vi "Begin.vi"() -> (0 "error out":errorcluster)   [LabVIEW 2011]
doc: "Called before other user functions, this VI is expected to open initial I/O refnums, load in file data, and do all program initialization. Notice that the <B>error out</B> terminal is simply used for data flow. Wiring it to other structures or subVIs ensures that this VI runs first."
uses:
  <vilib>/Rock Robotics/WPI/Joystick/WPI_JoystickDeviceEnum.ctl
  <vilib>/Rock Robotics/SystemInterfaces/DIO/FPGA_DIOChannel.ctl
  <vilib>/Rock Robotics/SystemInterfaces/Typedef/FPGA_TypedefDigitalModule.ctl
  <vilib>/Rock Robotics/SystemInterfaces/AI/FPGA_AIGyroChannel.ctl
  <vilib>/Rock Robotics/SystemInterfaces/DIO/FPGA_DIOPWMChannel.ctl
  <vilib>/Rock Robotics/SystemInterfaces/AI/FPGA_AIChannel.ctl
  <vilib>/Rock Robotics/SystemInterfaces/DIO/FPGA_DIORelayChannel.ctl
  <vilib>/Rock Robotics/SystemInterfaces/Typedef/FPGA_TypedefSolenoidModule.ctl
  <vilib>/Rock Robotics/WPI/Solenoid/WPI_SolenoidChannel.ctl
  <vilib>/Rock Robotics/WPI/Solenoid/WPI_SolenoidValue.ctl
  <vilib>/Rock Robotics/WPI/Relay/WPI_RelayDirection.ctl
  <vilib>/Rock Robotics/SystemInterfaces/Typedef/FPGA_TypedefAnalogModule.ctl
  <vilib>/Rock Robotics/WPI/Relay/WPI_RelayValue.ctl
  <vilib>/Rock Robotics/SystemInterfaces/Typedef/FPGA_TypedefAnalogModuleForGyro.ctl
  <vilib>/Rock Robotics/WPI/Counter/WPI_CounterOpen UpDown Mode.vi
  <vilib>/Rock Robotics/WPI/MotorControl/WPI_MotorControlOpen Victor.vi
  <vilib>/Rock Robotics/WPI/RobotDrive/WPI_RobotDriveOpen2MotorWithVictor.vi
  <vilib>/Rock Robotics/WPI/Solenoid/WPI_SolenoidSetEnum.vi
  <vilib>/Rock Robotics/WPI/Solenoid/WPI_SolenoidOpenDouble.vi
  Robot Global Data.vi
  <vilib>/Rock Robotics/WPI/Camera/WPI_CameraWhite Balance Values.ctl
  <vilib>/Rock Robotics/WPI/Camera/WPI_CameraExposure Values.ctl
  <vilib>/Rock Robotics/WPI/Camera/WPI_CameraFrameRate.ctl
  <vilib>/Rock Robotics/WPI/RobotDrive/WPI_RobotDriveOpen4MotorWithVictor.vi
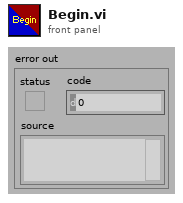
[diagram p1: front panel]
types:
  T1 = typedef "FPGA_AIGyroChannel.ctl" = enum8{"AI 1", "AI 2", "Invalid"}
  T2 = typedef "FPGA_TypedefAnalogModuleForGyro.ctl" = enum16{"Analog Module 1"}
  T3 = typedef "WPI_RelayDirection.ctl" = enum16{"Both directions", "Forward only", "Reverse only"}
  T4 = typedef "WPI_RelayValue.ctl" = enum16{"Off", "On", "Forward", "Reverse"}
  T5 = typedef "FPGA_DIORelayChannel.ctl" = enum8{"Relay 1", "Relay 2", "Relay 3", "Relay 4", "Relay 5", "Relay 6", "Relay 7", "Relay 8", "Invalid"}
  T6 = typedef "FPGA_TypedefDigitalModule.ctl" = enum16{"Digital Module 1", "Digital Module 2"}
  T7 = typedef "FPGA_AIChannel.ctl" = enum8{"AI 1", "AI 2", "AI 3", "AI 4", "AI 5", "AI 6", "AI 7", "AI 8", "Invalid"}
  T8 = typedef "FPGA_TypedefAnalogModule.ctl" = enum16{"Analog Module 1", "Analog Module 2"}
  T9 = typedef "FPGA_DIOPWMChannel.ctl" = enum8{"PWM 1", "PWM 2", "PWM 3", "PWM 4", "PWM 5", "PWM 6", "PWM 7", "PWM 8", "PWM 9", "PWM 10", "Invalid"}
  T10 = typedef "FPGA_DIOChannel.ctl" = enum8{"DIO 1", "DIO 2", "DIO 3", "DIO 4", "DIO 5", "DIO 6", "DIO 7", "DIO 8", "DIO 9", "DIO 10", "DIO 11", "DIO 12", "DIO 13", "DIO 14", "Invalid"}
  T11 = typedef "WPI_SolenoidValue.ctl" = enum16{"Off", "On", "Forward", "Reverse"}
  T12 = typedef "WPI_SolenoidChannel.ctl" = enum8{"Solenoid 1", "Solenoid 2", "Solenoid 3", "Solenoid 4", "Solenoid 5", "Solenoid 6", "Solenoid 7", "Solenoid 8", "Invalid"}
  T13 = typedef "FPGA_TypedefSolenoidModule.ctl" = enum16{"Solenoid Module 1", "Solenoid Module 2"}
  T14 = enum16{"Rising Edge", "Falling Edge", "Raising & Falling Edge", "Disabled"}
  T15 = typedef "WPI_JoystickDeviceEnum.ctl" = enum16{"USB 1", "USB 2", "USB 3", "USB 4", "Kinect 1", "Kinect 2"}
  T16 = typedef "WPI_CameraFrameRate.ctl" = u32
  T17 = typedef "WPI_CameraExposure Values.ctl" = enum16{"Auto", "Flicker-free 50 Hz", "Flicker-free 60 Hz", "Hold current"}
  T18 = typedef "WPI_CameraWhite Balance Values.ctl" = enum16{"Auto", "Fixed indoor", "Fixed outdoor 1", "Fixed outdoor 2", "Fixed fluorescent 1", "Fixed fluorescent 2", "Hold current"}
  T19 = typedef "WPI_CameraDevRef.ctl" = cluster{"Camera Address":string, "CameraStatus":errorcluster, "Acquire Image Notifier":refnum<notifier>}
  T20 = typedef "WPI_CameraImageSize.ctl" = enum16{"640x480", "320x240", "160x120"}
  T21 = typedef "WPI_RelayDevRef.ctl" = cluster{"DevStatus":errorcluster, "Relay Channel":T5, "Digital Module":T6, "Relay Direction":T3}
  T22 = typedef "WPI_AccelerometerDevRef.ctl" = cluster{"DevStatus":errorcluster, "Analog Module":T8, "Analog Channel":T7, "Scaling":T23}
  T23 = typedef "WPI_AccelerometerScaling.ctl" = cluster{"Gain (VoltsPerG)":dbl, "Center Voltage":dbl}
  T24 = typedef "WPI_DigitalInputDevRef.ctl" = cluster{"DevStatus":errorcluster, "DIO Channel":T10, "Digital Module":T6}
  T25 = typedef "WPI_RobotDriveDevRef.ctl" = cluster{"DevStatus":errorcluster, "Motors[]":T26[], "Square Inputs":bool, "Max Output":dbl, "Isochronous":bool}
  T26 = typedef "WPI_MotorControlDeviceRef.ctl" = cluster{"DeviceStatus":errorcluster, "Type":enum16{"PWM", "CAN"}, "PWM":cluster{"Digital Module":T6, "PWM Channel":T9, "DeadBand":T27}, "CAN":cluster{"Device Number":u8, "Control Mode":T28, "Semaphore":T29, "Max Vout":dbl}, "Invert":bool, "TransformRef":T30, "InvTransformRef":T30}
  T27 = typedef "WPI_PWMDeadband.ctl" = cluster{"Name":string, "maxPositivePwm":i32, "minPositivePwm":i32, "centerPwm":i32, "maxNegativePwm":i32, "minNegativePwm":i32, "angularRange":u16}
  T28 = typedef "WPI_CANJaguar_ControlMode.ctl" = enum8{"Percent VBus", "Current", "Speed", "Position", "Voltage"}
  T29 = typedef "Semaphore RefNum" = refnum<k1>
  T30 = typedef "WPI_PWMTransform_ConPane.ctl" = refnum<vi>
  T31 = typedef "WPI_JoystickDevRef.ctl" = cluster{"Device":T15}
  T32 = typedef "FPGA_CounterEncoderSourceConvertionLVSourceType.ctl" = cluster{"DevStatus":errorcluster, "AnalogTriggerMode?":bool, "DigitalMode":cluster{"Digital Module":T6, "DIO Channel":T33}, "AnalogTriggerMode":cluster{"AnalogTriggerIndex":T34, "OutputType":T35}}
  T33 = typedef "FPGA_DIODigitalSourceChannel.ctl" = enum8{"DIO 1", "DIO 2", "DIO 3", "DIO 4", "DIO 5", "DIO 6", "DIO 7", "DIO 8", "DIO 9", "DIO 10", "DIO 11", "DIO 12", "DIO 13", "DIO 14", "Disabled"}
  T34 = typedef "FPGA_AnalogTriggerIndex.ctl" = enum8{"Trig 0", "Trig 1", "Trig 2", "Trig 3", "Trig 4", "Trig 5", "Trig 6", "Trig 7", "Invalid"}
  T35 = typedef "FPGA_AnalogTriggerOutType.ctl" = enum16{"InWindow", "TriggerState", "Rising", "Falling"}
  T36 = typedef "WPI_AnalogChannelDevRef.ctl" = cluster{"DevStatus":errorcluster, "Analog Module":T8, "Analog Channel":T7}
  T37 = typedef "WPI_GyroDevRef.ctl" = cluster{"DevStatus":errorcluster, "Analog Module":T8, "Analog Channel":T7, "Offset":dbl, "Gain (VoltsPerDegree/Second)":dbl}
  T38 = typedef "WPI_SolenoidDevRef.ctl" = cluster{"DevStatus":errorcluster, "Solenoid Module":T13, "Forward Solenoid Channel":T12, "Reverse Solenoid Channel":T12}
  T39 = typedef "WPI_CounterDevRef.ctl" = cluster{"DevStatus":errorcluster, "CntIndex":T40}
  T40 = typedef "FPGA_CounterCtrSystemIndex.ctl" = enum8{"Ctr 0", "Ctr 1", "Ctr 2", "Ctr 3", "Ctr 4", "Ctr 5", "Ctr 6", "Ctr 7", "Invalid"}
  T41 = typedef "WPI_EncoderDevRef.ctl" = cluster{"DevStatus":errorcluster, "EncoderIndex":T42, "CounterIndex":T40, "DistancePerCount":dbl, "Decoding Type":T43}
  T42 = typedef "FPGA_EncoderIdx.ctl" = enum8{"Enc 0", "Enc 1", "Enc 2", "Enc 3", "Invalid"}
  T43 = typedef "WPI_EncoderType.ctl" = enum16{"1x", "2x", "4x"}
  T44 = typedef "WPI_ServoDeviceRef.ctl" = cluster{"DeviceStatus":errorcluster, "Digital Module":T6, "PWM Channel":T9, "DeadBand":T27}
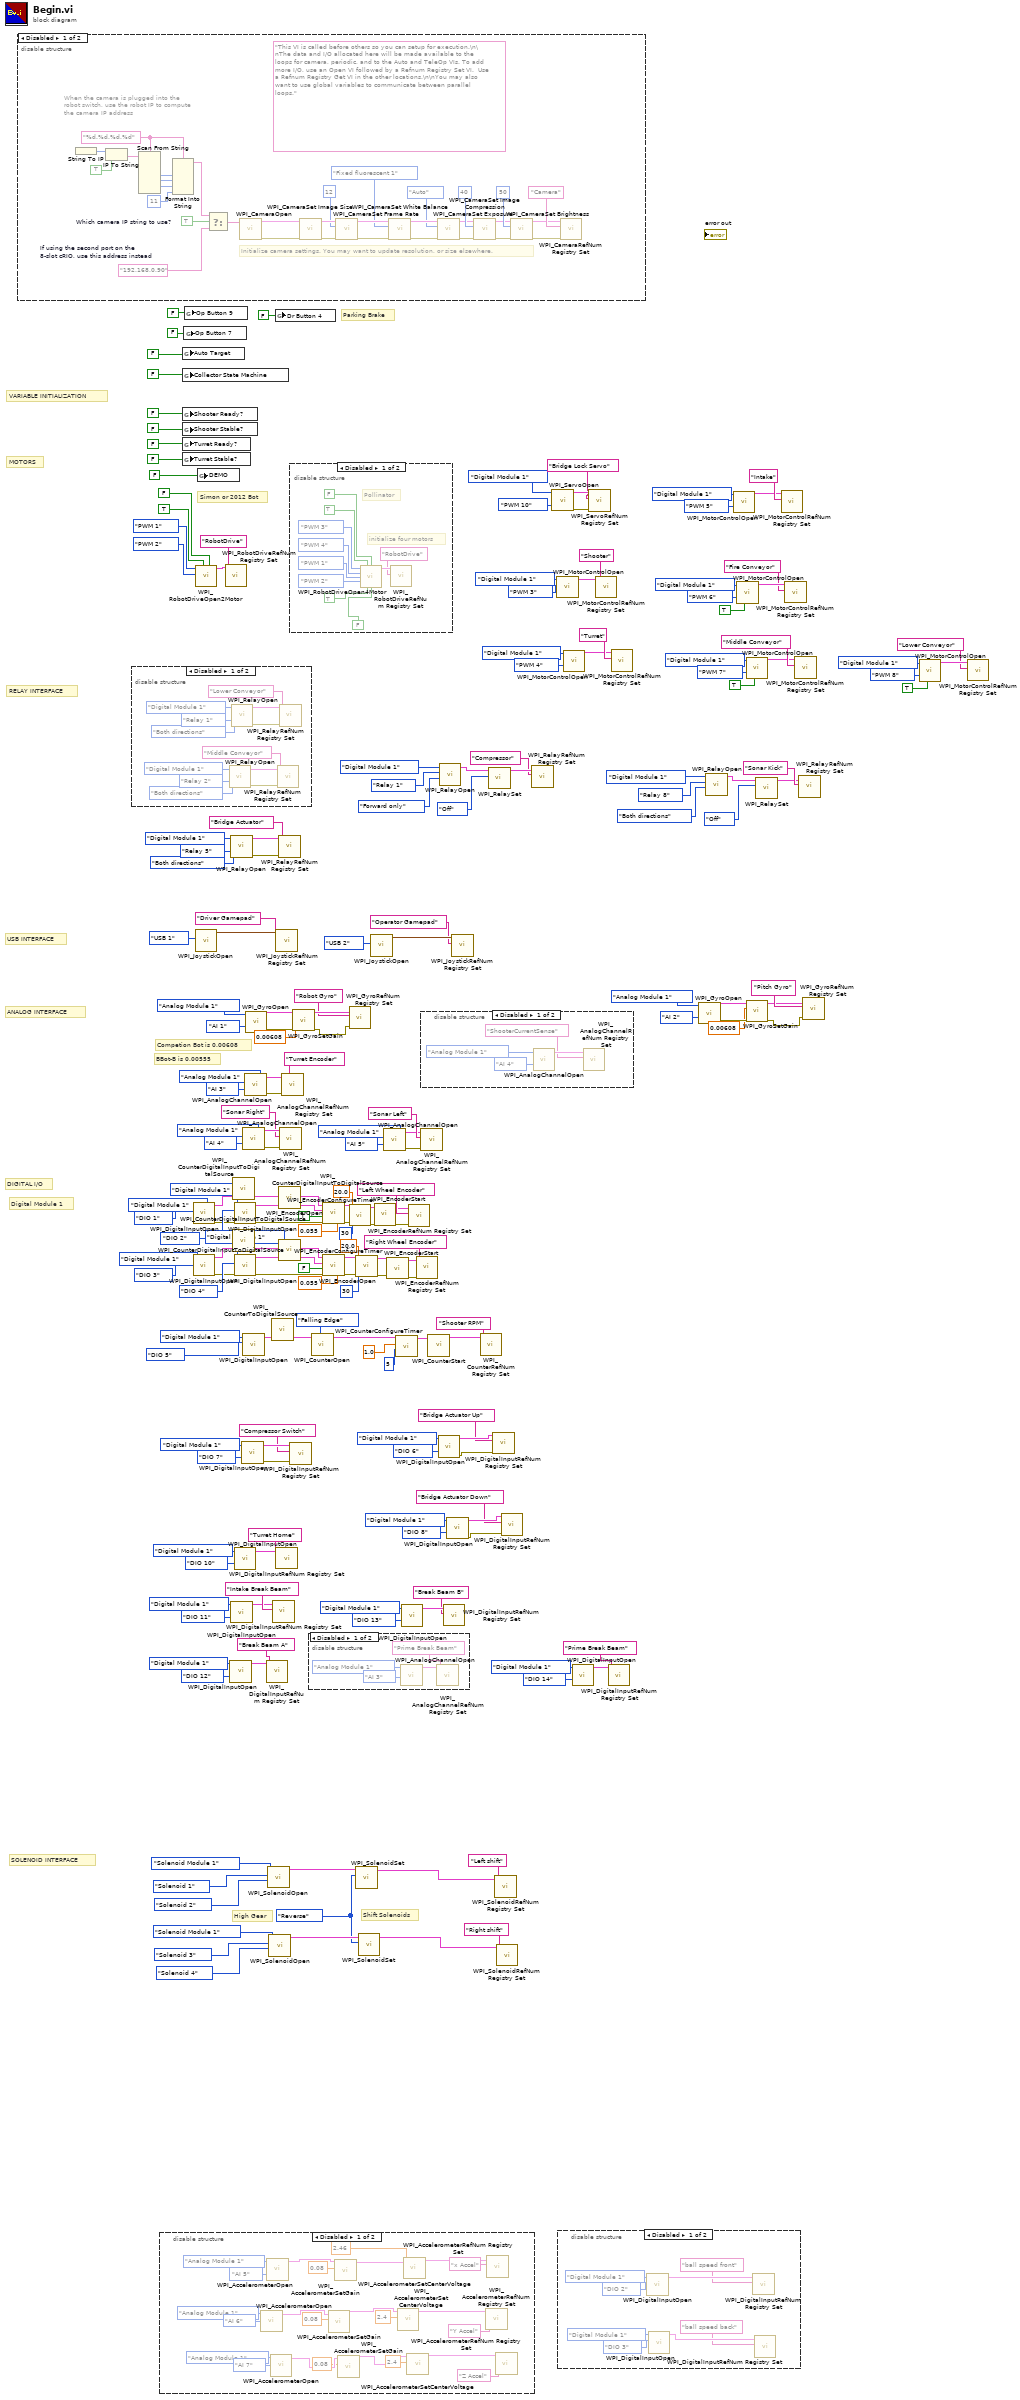
[diagram p0: block diagram]
diagram:
  w79 = WPI_SolenoidValue."Reverse" ("Value")
  # "Parking Brake"
  # "BBot-B is 0.00555"
  # "Competion Bot is 0.00608"
  # "Digital Module 1"
  # "SOLENOID INTERFACE"
  # "High Gear"
  # "Shift Solenoids"
  # "Simon or 2012 Bot"
  # "RELAY INTERFACE"
  # "MOTORS"
  # "VARIABLE INITIALIZATION"
  # "DIGITAL I/O"
  # "USB INTERFACE"
  # "ANALOG INTERFACE"
  n1 = disable-structure shown="Disabled" {
    frame Disabled {
      w207 = TRUE  # Which camera IP string to use?
      w211 = "%d.%d.%d.%d" ("format string")
      (unwired) "This VI is called before others so you can setup for execution.\n\nThe data and I/O allocated here will be made available to the loops for camera, periodic, and to the Auto and TeleOp VIs. To add more I/O, use an Open VI followed by a Refnum Registry Set VI.  Use a Refnum Registry Get VI in the other locations.\n\nYou may also want to use global variables to communicate between parallel loops."
      w208 = "192.168.0.90"  # If using the second port on the 8-slot cRIO, use this address instead
      # "When the camera is plugged into the\nrobot switch, use the robot IP to compute\nthe camera IP address"
      # "Initialize camera settings. You may want to update resolution, or size elsewhere."
      n2 = String To IP() -> (0:w218:u32)  [unwired: 1 in]
      n3 = IP To String(1:TRUE ("dot notation? (F)"), 2:w218) -> (0:w216:string)
      n4 = Scan From String(format string=w211, input string=w216) -> (output 1=w215:i32, output 2=w214:i32, output 3=w213:i32)  [unwired: 7 in, 3 out]
      n5 = Format Into String(format string=w211, w215, w214, w213, 11 ("Compression")) -> (resulting string=w209:string)  [unwired: 2 in, 1 out]
      n6 = Select(t=w209, s=w207, f=w208) -> (s? t:f=w210:string)
      n7 = call <vilib>:"WPI_CameraOpen.vi"("Camera Address"=w210) -> ("error out"=w230:errorcluster, "CameraDevRef"=w231:T19)  [unwired: 1 in, 8 out]
      n8 = call <vilib>:"WPI_CameraSet Image Size.vi"("error in (no error)"=w230, "CameraDevRef"=w231) -> ("error out"=w229:errorcluster, "CameraDevRef Out"=w232:T19, "Image Size"=w222:T20)  [unwired: 7 out]
      n9 = call <vilib>:"WPI_CameraSet Frame Rate.vi"("error in (no error)"=w229, "Frame Rate (fps)"=T16 12, "CameraDevRef"=w232) -> ("error out"=w228:errorcluster, "CameraDevRef Out"=w234:T19)  [unwired: 7 out]
      n10 = call <vilib>:"WPI_CameraSet White Balance.vi"("error in (no error)"=w228, "White Balance"=WPI_CameraWhite_Balance_Values."Fixed fluorescent 1", "CameraDevRef"=w234) -> ("error out"=w227:errorcluster, "CameraDevRef Out"=w233:T19)  [unwired: 7 out]
      n11 = call <vilib>:"WPI_CameraSet Exposure.vi"("error in (no error)"=w227, "Exposure"=WPI_CameraExposure_Values."Auto", "CameraDevRef"=w233) -> ("error out"=w226:errorcluster, "CameraDevRef Out"=w236:T19)  [unwired: 7 out]
      n12 = call <vilib>:"WPI_CameraSet Image Compression.vi"("error in (no error)"=w226, "Compression"=40, "CameraDevRef"=w236) -> ("error out"=w225:errorcluster, "CameraDevRef Out"=w235:T19)  [unwired: 7 out]
      n13 = call <vilib>:"WPI_CameraSet Brightness.vi"("error in (no error)"=w225, "Brightness"=50, "CameraDevRef"=w235) -> ("error out"=w223:errorcluster, "CameraDevRef Out"=w224:T19)  [unwired: 7 out]
      n14 = call <vilib>:"WPI_CameraRefNum Registry Set.vi"("error in (no error)"=w223, "refnum name"="Camera", "CameraDevRef"=w224) -> ()  [unwired: 9 out]
    }
    frame Enabled {
    }
  }
  n15 = disable-structure shown="Disabled" {
    frame Disabled {
      n16 = call <vilib>:"WPI_RelayOpen.vi"("Relay Direction"=WPI_RelayDirection."Both directions", "Relay Channel"=FPGA_DIORelayChannel."Relay 2", "Digital Module (Module 1)"=FPGA_TypedefDigitalModule."Digital Module 1") -> ("error out"=w250:errorcluster, "RelayDevRef"=w249:T21)  [unwired: 7 in]
      n17 = call <vilib>:"WPI_RelayOpen.vi"("Relay Direction"=WPI_RelayDirection."Both directions", "Relay Channel"=FPGA_DIORelayChannel."Relay 1", "Digital Module (Module 1)"=FPGA_TypedefDigitalModule."Digital Module 1") -> ("error out"=w241:errorcluster, "RelayDevRef"=w242:T21)  [unwired: 7 in]
      n18 = call <vilib>:"WPI_RelayRefNum Registry Set.vi"("error in (no error)"=w250, "refnum name"="Middle Conveyor", "RelayDevRef"=w249) -> ()  [unwired: 7 in, 2 out]
      n19 = call <vilib>:"WPI_RelayRefNum Registry Set.vi"("error in (no error)"=w241, "refnum name"="Lower Conveyor", "RelayDevRef"=w242) -> ()  [unwired: 7 in, 2 out]
    }
    frame Enabled {
    }
  }
  n20 = disable-structure shown="Disabled" {
    frame Disabled {
      n21 = call <vilib>:"WPI_AccelerometerOpen.vi"("Analog Channel"=FPGA_AIChannel."AI 6", "Analog Module (Module 1)"=FPGA_TypedefAnalogModule."Analog Module 1") -> ("AccelerometerDevRef"=w258:T22)  [unwired: 8 in, 1 out]
      n22 = call <vilib>:"WPI_AccelerometerOpen.vi"("Analog Channel"=FPGA_AIChannel."AI 5", "Analog Module (Module 1)"=FPGA_TypedefAnalogModule."Analog Module 1") -> ("AccelerometerDevRef"=w259:T22)  [unwired: 8 in, 1 out]
      n23 = call <vilib>:"WPI_AccelerometerOpen.vi"("Analog Channel"=FPGA_AIChannel."AI 7", "Analog Module (Module 1)"=FPGA_TypedefAnalogModule."Analog Module 1") -> ("AccelerometerDevRef"=w272:T22)  [unwired: 8 in, 1 out]
      n24 = call <vilib>:"WPI_AccelerometerSetGain.vi"("Gain (VoltsPerG)"=0.08, "AccelerometerDevRef"=w258) -> ("AccelerometerDevRef"=w257:T22)  [unwired: 8 in, 1 out]
      n25 = call <vilib>:"WPI_AccelerometerSetGain.vi"("Gain (VoltsPerG)"=0.08, "AccelerometerDevRef"=w259) -> ("AccelerometerDevRef"=w260:T22)  [unwired: 8 in, 1 out]
      n26 = call <vilib>:"WPI_AccelerometerSetGain.vi"("Gain (VoltsPerG)"=0.08, "AccelerometerDevRef"=w272) -> ("AccelerometerDevRef"=w271:T22)  [unwired: 8 in, 1 out]
      n27 = call <vilib>:"WPI_AccelerometerSetCenterVoltage.vi"("Center Voltage"=2.4, "AccelerometerDevRef"=w257) -> ("AccelerometerDevRef"=w256:T22)  [unwired: 8 in, 1 out]
      n28 = call <vilib>:"WPI_AccelerometerSetCenterVoltage.vi"("Center Voltage"=2.46, "AccelerometerDevRef"=w260) -> ("AccelerometerDevRef"=w261:T22)  [unwired: 8 in, 1 out]
      n29 = call <vilib>:"WPI_AccelerometerSetCenterVoltage.vi"("Center Voltage"=2.4, "AccelerometerDevRef"=w271) -> ("AccelerometerDevRef"=w270:T22)  [unwired: 8 in, 1 out]
      n30 = call <vilib>:"WPI_AccelerometerRefNum Registry Set.vi"("refnum name"="Y Accel", "AccelerometerDevRef"=w256) -> ()  [unwired: 8 in, 2 out]
      n31 = call <vilib>:"WPI_AccelerometerRefNum Registry Set.vi"("refnum name"="x Accel", "AccelerometerDevRef"=w261) -> ()  [unwired: 8 in, 2 out]
      n32 = call <vilib>:"WPI_AccelerometerRefNum Registry Set.vi"("refnum name"="Z Accel", "AccelerometerDevRef"=w270) -> ()  [unwired: 8 in, 2 out]
    }
    frame Enabled {
    }
  }
  n33 = global write "Robot Global Data.vi" "Auto Target"(FALSE ("Auto Target")) -> ()
  n34 = global write "Robot Global Data.vi" "Collector State Machine"(FALSE ("Shooter Ready?")) -> ()
  n35 = global write "Robot Global Data.vi" "Shooter Ready?"(FALSE ("Shooter Ready?")) -> ()
  n36 = global write "Robot Global Data.vi" "Shooter Stable?"(FALSE ("Shooter Stable?")) -> ()
  n37 = global write "Robot Global Data.vi" "Turret Ready?"(FALSE ("Turret Ready?")) -> ()
  n38 = global write "Robot Global Data.vi" "Turret Stable?"(FALSE ("Turret Stable?")) -> ()
  n39 = global write "Robot Global Data.vi" "Op Button 7"(FALSE ("Op Button 9")) -> ()
  n40 = global write "Robot Global Data.vi" "Op Button 9"(FALSE ("Op Button 9")) -> ()
  n41 = call <vilib>:"WPI_DigitalInputOpen.vi"("DIO Channel"=FPGA_DIOChannel."DIO 1", "Digital Module (Module 1)"=FPGA_TypedefDigitalModule."Digital Module 1" ("DIO Module (Slot 4)")) -> ("error out"=w193:errorcluster, "DigitalInputDevRef"=w198:T24)  [unwired: 1 in, 7 out]
  n42 = call <vilib>:"WPI_DigitalInputOpen.vi"("DIO Channel"=FPGA_DIOChannel."DIO 3", "Digital Module (Module 1)"=FPGA_TypedefDigitalModule."Digital Module 1" ("DIO Module (Slot 4)")) -> ("error out"=w185:errorcluster, "DigitalInputDevRef"=w190:T24)  [unwired: 1 in, 7 out]
  n43 = call-poly <vilib>:"WPI_RobotDriveOpen2Motor.vi"("Right Motor Inverted"=FALSE ("Rear Right Motor Inverted"), "Left Motor Inverted"=TRUE ("Rear Left Motor Inverted"), "Right Motor"=FPGA_DIOPWMChannel."PWM 2" ("Rear Right Motor"), "Left Motor"=FPGA_DIOPWMChannel."PWM 1" ("Rear Left Motor")) -> ("RobotDriveDevRef"=w119:T25)  [unwired: 6 in, 1 out]
  n44 = call <vilib>:"WPI_JoystickOpen.vi"("JoystickDevice"=WPI_JoystickDeviceEnum."USB 1") -> ("JoystickDevRef"=w203:T31)  [unwired: 10 out]
  n45 = global write "Robot Global Data.vi" "DEMO"(FALSE ("Turret Stable?")) -> ()
  n46 = call <vilib>:"WPI_RobotDriveRefNum Registry Set.vi"("refnum name"="RobotDrive", "RobotDriveDevRef"=w119) -> ()  [unwired: 1 in, 9 out]
  n47 = call <vilib>:"WPI_DigitalInputOpen.vi"("DIO Channel"=FPGA_DIOChannel."DIO 12", "Digital Module (Module 1)"=FPGA_TypedefDigitalModule."Digital Module 1") -> ("DigitalInputDevRef"=w114:T24)  [unwired: 8 in, 1 out]
  n48 = call <vilib>:"WPI_RelayOpen.vi"("Relay Direction"=WPI_RelayDirection."Both directions", "Relay Channel"=FPGA_DIORelayChannel."Relay 5", "Digital Module (Module 1)"=FPGA_TypedefDigitalModule."Digital Module 1") -> ("error out"=w94:errorcluster, "RelayDevRef"=w95:T21)  [unwired: 7 in]
  n49 = call <vilib>:"WPI_DigitalInputOpen.vi"("DIO Channel"=FPGA_DIOChannel."DIO 11", "Digital Module (Module 1)"=FPGA_TypedefDigitalModule."Digital Module 1") -> ("DigitalInputDevRef"=w110:T24)  [unwired: 8 in, 1 out]
  n50 = call <vilib>:"WPI_CounterDigitalInputToDigitalSource.vi"("DigitalInputDevRef"=w198) -> ("Digital Source"=w197:T32)  [unwired: 6 out]
  n51 = call <vilib>:"WPI_CounterDigitalInputToDigitalSource.vi"("DigitalInputDevRef"=w190) -> ("Digital Source"=w189:T32)  [unwired: 6 out]
  n52 = call <vilib>:"WPI_DigitalInputOpen.vi"("error in (no error)"=w193, "DIO Channel"=FPGA_DIOChannel."DIO 2", "Digital Module (Module 1)"=FPGA_TypedefDigitalModule."Digital Module 1" ("DIO Module (Slot 4)")) -> ("error out"=w194:errorcluster, "DigitalInputDevRef"=w196:T24)  [unwired: 7 out]
  n53 = call <vilib>:"WPI_DigitalInputOpen.vi"("error in (no error)"=w185, "DIO Channel"=FPGA_DIOChannel."DIO 4", "Digital Module (Module 1)"=FPGA_TypedefDigitalModule."Digital Module 1" ("DIO Module (Slot 4)")) -> ("error out"=w186:errorcluster, "DigitalInputDevRef"=w188:T24)  [unwired: 7 out]
  n54 = call <vilib>:"WPI_DigitalInputOpen.vi"("DIO Channel"=FPGA_DIOChannel."DIO 10", "Digital Module (Module 1)"=FPGA_TypedefDigitalModule."Digital Module 1") -> ("DigitalInputDevRef"=w72:T24)  [unwired: 8 in, 1 out]
  n55 = call <vilib>:"WPI_DigitalInputOpen.vi"("DIO Channel"=FPGA_DIOChannel."DIO 7", "Digital Module (Module 1)"=FPGA_TypedefDigitalModule."Digital Module 1") -> ("error out"=w64:errorcluster, "DigitalInputDevRef"=w65:T24)  [unwired: 8 in]
  n56 = call <vilib>:"WPI_AnalogChannelOpen.vi"("Analog Channel"=FPGA_AIChannel."AI 4", "Analog Module (Module 1)"=FPGA_TypedefAnalogModule."Analog Module 1" ("Analog Module (Slot 1)")) -> ("error out"=w22:errorcluster, "AIDeviceRef"=w23:T36)  [unwired: 1 in, 7 out]
  n57 = call <vilib>:"WPI_DigitalInputOpen.vi"("DIO Channel"=FPGA_DIOChannel."DIO 5", "Digital Module (Module 1)"=FPGA_TypedefDigitalModule."Digital Module 1") -> ("DigitalInputDevRef"=w148:T24)  [unwired: 8 in, 1 out]
  n58 = call <vilib>:"WPI_AnalogChannelOpen.vi"("Analog Channel"=FPGA_AIChannel."AI 3", "Analog Module (Module 1)"=FPGA_TypedefAnalogModule."Analog Module 1" ("Analog Module (Slot 1)")) -> ("error out"=w103:errorcluster, "AIDeviceRef"=w102:T36)  [unwired: 1 in, 7 out]
  n59 = call <vilib>:"WPI_GyroOpen.vi"("Analog Channel"=FPGA_AIGyroChannel."AI 1", "Analog Module (Module 1)"=FPGA_TypedefAnalogModuleForGyro."Analog Module 1") -> ("error out"=w152:errorcluster, "GyroDevRef"=w157:T37)  [unwired: 7 in, 1 out]
  n60 = call <vilib>:"WPI_DigitalInputRefNum Registry Set.vi"("refnum name"="Break Beam A", "DigitalInputDevRef"=w114) -> ()  [unwired: 8 in, 2 out]
  n61 = call-poly <vilib>:"WPI_SolenoidOpen.vi"("Reverse Solenoid Channel"=WPI_SolenoidChannel."Solenoid 2", "Forward Solenoid Channel"=WPI_SolenoidChannel."Solenoid 1", "Solenoid Module (Module 1)"=FPGA_TypedefSolenoidModule."Solenoid Module 1") -> ("SolenoidDevRef"=w83:T38)  [unwired: 7 in, 1 out]
  n62 = call-poly <vilib>:"WPI_SolenoidOpen.vi"("Reverse Solenoid Channel"=WPI_SolenoidChannel."Solenoid 4", "Forward Solenoid Channel"=WPI_SolenoidChannel."Solenoid 3", "Solenoid Module (Module 1)"=FPGA_TypedefSolenoidModule."Solenoid Module 1") -> ("SolenoidDevRef"=w81:T38)  [unwired: 7 in, 1 out]
  n63 = call-poly <vilib>:"WPI_CounterToDigitalSource.vi"("DigitalInputDevRef"=w148) -> ("Digital Source"=w147:T32)  [unwired: 6 in]
  n64 = call <vilib>:"WPI_DigitalInputRefNum Registry Set.vi"("refnum name"="Intake Break Beam", "DigitalInputDevRef"=w110) -> ()  [unwired: 8 in, 2 out]
  n65 = global write "Robot Global Data.vi" "Dr Button 4"(FALSE ("Dr Button 4")) -> ()
  n66 = call <vilib>:"WPI_JoystickRefNum Registry Set.vi"("refnum name"="Driver Gamepad", "JoystickDevRef"=w203) -> ()  [unwired: 1 in, 9 out]
  n67 = call <vilib>:"WPI_DigitalInputRefNum Registry Set.vi"("refnum name"="Turret Home", "DigitalInputDevRef"=w72) -> ()  [unwired: 8 in, 2 out]
  n68 = call <vilib>:"WPI_RelayRefNum Registry Set.vi"("error in (no error)"=w94, "refnum name"="Bridge Actuator", "RelayDevRef"=w95) -> ()  [unwired: 7 in, 2 out]
  n69 = call <vilib>:"WPI_CounterDigitalInputToDigitalSource.vi"("DigitalInputDevRef"=w196) -> ("Digital Source"=w195:T32)  [unwired: 6 out]
  n70 = call <vilib>:"WPI_CounterDigitalInputToDigitalSource.vi"("DigitalInputDevRef"=w188) -> ("Digital Source"=w187:T32)  [unwired: 6 out]
  n71 = call <vilib>:"WPI_AnalogChannelRefNum Registry Set.vi"("error in (no error)"=w22, "refnum name"="Sonar Right", "AIDeviceRef"=w23) -> ()  [unwired: 9 out]
  n72 = call <vilib>:"WPI_AnalogChannelRefNum Registry Set.vi"("error in (no error)"=w103, "refnum name"="Turret Encoder", "AIDeviceRef"=w102) -> ()  [unwired: 9 out]
  n73 = disable-structure shown="Disabled" {
    frame Disabled {
      # "initialize four motors"
      # "Pollinator"
      n74 = call-poly <vilib>:"WPI_RobotDriveOpen4Motor.vi"("Rear Left Motor"=FPGA_DIOPWMChannel."PWM 3", "Rear Left Motor Inverted"=TRUE, "Rear Right Motor Inverted"=FALSE, "Rear Right Motor"=FPGA_DIOPWMChannel."PWM 4", "Front Left Motor"=FPGA_DIOPWMChannel."PWM 1", "Front Right Motor"=FPGA_DIOPWMChannel."PWM 2", "Front Left Motor Inverted"=TRUE, "Front Right Motor Inverted"=FALSE) -> ("RobotDriveDevRef"=w279:T25)  [unwired: 1 in, 6 out]
      n75 = call <vilib>:"WPI_RobotDriveRefNum Registry Set.vi"("refnum name"="RobotDrive", "RobotDriveDevRef"=w279) -> ()  [unwired: 1 in, 9 out]
    }
    frame Enabled {
    }
  }
  n76 = call <vilib>:"WPI_DigitalInputRefNum Registry Set.vi"("error in (no error)"=w64, "refnum name"="Compressor Switch", "DigitalInputDevRef"=w65) -> ()  [unwired: 7 in, 2 out]
  n77 = call <vilib>:"WPI_GyroSetGain.vi"("error in (no error)"=w152, "Gain (VoltsPerDegree/Second)"=0.00608, "GyroDevRef"=w157) -> ("error out"=w153:errorcluster, "GyroDevRef"=w155:T37)  [unwired: 7 in]
  n78 = disable-structure shown="Disabled" {
    frame Disabled {
      n79 = call <vilib>:"WPI_AnalogChannelOpen.vi"("Analog Channel"=FPGA_AIChannel."AI 3", "Analog Module (Module 1)"=FPGA_TypedefAnalogModule."Analog Module 1") -> ("AIDeviceRef"=w286:T36)  [unwired: 8 in, 1 out]
      n80 = call <vilib>:"WPI_AnalogChannelRefNum Registry Set.vi"("refnum name"="Prime Break Beam", "AIDeviceRef"=w286) -> ()  [unwired: 8 in, 2 out]
    }
    frame Enabled {
    }
  }
  n81 = call-poly <vilib>:"WPI_CounterOpen.vi"("UpEdge"=T14."Falling Edge", "Up Source"=w147) -> ("CounterDevRef"=w132:T39)  [unwired: 8 in, 1 out]
  n82 = call <vilib>:"WPI_EncoderOpen.vi"("DistancePerCount"=0.055, "error in (no error)"=w194, "Invert Direction (False)"=TRUE, "BSource"=w195, "ASource"=w197) -> ("error out"=w174:errorcluster, "EncoderDevRef"=w175:T41)  [unwired: 3 in, 2 out]
  n83 = call <vilib>:"WPI_EncoderOpen.vi"("DistancePerCount"=0.055, "error in (no error)"=w186, "Invert Direction (False)"=FALSE, "BSource"=w187, "ASource"=w189) -> ("error out"=w170:errorcluster, "EncoderDevRef"=w171:T41)  [unwired: 3 in, 2 out]
  n84 = call <vilib>:"WPI_GyroRefNum Registry Set.vi"("error in (no error)"=w153, "refnum name"="Robot Gyro", "GyroDevRef"=w155) -> ()  [unwired: 7 in, 2 out]
  n85 = call <vilib>:"WPI_EncoderConfigureTimer.vi"("error in (no error)"=w174, "Number Samples to Average"=u8 30, "Minimum Rate"=20.0, "EncoderDevRef"=w175) -> ("error out"=w172:errorcluster, "EncoderDevRef"=w173:T41)  [unwired: 6 out]
  n86 = call <vilib>:"WPI_EncoderConfigureTimer.vi"("error in (no error)"=w170, "Number Samples to Average"=u8 30, "Minimum Rate"=20.0, "EncoderDevRef"=w171) -> ("error out"=w168:errorcluster, "EncoderDevRef"=w169:T41)  [unwired: 6 out]
  n87 = call-poly <vilib>:"WPI_SolenoidSet.vi"("Value"=w79, "SolenoidDevRef"=w83) -> ("SolenoidDevRef"=w82:T38)  [unwired: 8 in, 1 out]
  n88 = call-poly <vilib>:"WPI_SolenoidSet.vi"("Value"=w79, "SolenoidDevRef"=w81) -> ("SolenoidDevRef"=w80:T38)  [unwired: 8 in, 1 out]
  n89 = call <vilib>:"WPI_JoystickOpen.vi"("JoystickDevice"=WPI_JoystickDeviceEnum."USB 2") -> ("JoystickDevRef"=w206:T31)  [unwired: 10 out]
  n90 = call <vilib>:"WPI_EncoderStart.vi"("error in (no error)"=w172, "EncoderDevRef"=w173) -> ("error out"=w182:errorcluster, "EncoderDevRef"=w183:T41)  [unwired: 8 out]
  n91 = call <vilib>:"WPI_AnalogChannelOpen.vi"("Analog Channel"=FPGA_AIChannel."AI 5", "Analog Module (Module 1)"=FPGA_TypedefAnalogModule."Analog Module 1" ("Analog Module (Slot 1)")) -> ("error out"=w19:errorcluster, "AIDeviceRef"=w18:T36)  [unwired: 1 in, 7 out]
  n92 = call <vilib>:"WPI_EncoderStart.vi"("error in (no error)"=w168, "EncoderDevRef"=w169) -> ("error out"=w176:errorcluster, "EncoderDevRef"=w181:T41)  [unwired: 8 out]
  n93 = call <vilib>:"WPI_CounterConfigureTimer.vi"("Number Samples to Average"=u8 5, "MaxPeriod (sec)"=1.0, "CounterDevRef in"=w132) -> ("CounterDevRef out"=w134:T39)  [unwired: 7 in, 1 out]
  n94 = call <vilib>:"WPI_DigitalInputOpen.vi"("DIO Channel"=FPGA_DIOChannel."DIO 13", "Digital Module (Module 1)"=FPGA_TypedefDigitalModule."Digital Module 1") -> ("DigitalInputDevRef"=w105:T24)  [unwired: 8 in, 1 out]
  n95 = call <vilib>:"WPI_EncoderRefNum Registry Set.vi"("error in (no error)"=w182, "refnum name"="Left Wheel Encoder", "EncoderDevRef"=w183) -> ()  [unwired: 9 out]
  n96 = call <vilib>:"WPI_EncoderRefNum Registry Set.vi"("error in (no error)"=w176, "refnum name"="Right Wheel Encoder", "EncoderDevRef"=w181) -> ()  [unwired: 9 out]
  n97 = disable-structure shown="Disabled" {
    frame Disabled {
      n98 = call <vilib>:"WPI_AnalogChannelOpen.vi"("Analog Channel"=FPGA_AIChannel."AI 4", "Analog Module (Module 1)"=FPGA_TypedefAnalogModule."Analog Module 1") -> ("AIDeviceRef"=w293:T36)  [unwired: 8 in, 1 out]
      n99 = call <vilib>:"WPI_AnalogChannelRefNum Registry Set.vi"("refnum name"="ShooterCurrentSense", "AIDeviceRef"=w293) -> ()  [unwired: 8 in, 2 out]
    }
    frame Enabled {
    }
  }
  n100 = call <vilib>:"WPI_AnalogChannelRefNum Registry Set.vi"("error in (no error)"=w19, "refnum name"="Sonar Left", "AIDeviceRef"=w18) -> ()  [unwired: 9 out]
  n101 = call <vilib>:"WPI_CounterStart.vi"("CounterDevRef in"=w134) -> ("CounterDevRef out"=w131:T39)  [unwired: 9 in, 1 out]
  n102 = call <vilib>:"WPI_DigitalInputOpen.vi"("DIO Channel"=FPGA_DIOChannel."DIO 6", "Digital Module (Module 1)"=FPGA_TypedefDigitalModule."Digital Module 1") -> ("error out"=w41:errorcluster, "DigitalInputDevRef"=w43:T24)  [unwired: 8 in]
  n103 = call <vilib>:"WPI_RelayOpen.vi"("Relay Direction"=WPI_RelayDirection."Forward only", "Relay Channel"=FPGA_DIORelayChannel."Relay 1", "Digital Module (Module 1)"=FPGA_TypedefDigitalModule."Digital Module 1" ("Relay Digital Module (Module 1)")) -> ("RelayDevRef"=w52:T21)  [unwired: 7 in, 1 out]
  n104 = call <vilib>:"WPI_DigitalInputRefNum Registry Set.vi"("refnum name"="Break Beam B", "DigitalInputDevRef"=w105) -> ()  [unwired: 8 in, 2 out]
  n105 = call <vilib>:"WPI_DigitalInputOpen.vi"("DIO Channel"=FPGA_DIOChannel."DIO 8", "Digital Module (Module 1)"=FPGA_TypedefDigitalModule."Digital Module 1") -> ("error out"=w36:errorcluster, "DigitalInputDevRef"=w38:T24)  [unwired: 8 in]
  n106 = call <vilib>:"WPI_JoystickRefNum Registry Set.vi"("refnum name"="Operator Gamepad", "JoystickDevRef"=w206) -> ()  [unwired: 1 in, 9 out]
  n107 = call <vilib>:"WPI_CounterRefNum Registry Set.vi"("refnum name"="Shooter RPM", "CounterDevRef"=w131) -> ()  [unwired: 8 in, 2 out]
  n108 = call <vilib>:"WPI_RelaySet.vi"("RelayValue"=WPI_RelayValue."Off", "RelayDevRef"=w52) -> ("RelayDevRef"=w51:T21)  [unwired: 8 in, 1 out]
  n109 = call <vilib>:"WPI_DigitalInputRefNum Registry Set.vi"("error in (no error)"=w41, "refnum name"="Bridge Actuator Up", "DigitalInputDevRef"=w43) -> ()  [unwired: 7 in, 2 out]
  n110 = call <vilib>:"WPI_SolenoidRefNum Registry Set.vi"("refnum name"="Left shift", "SolenoidDevRef"=w82) -> ()  [unwired: 8 in, 2 out]
  n111 = call <vilib>:"WPI_SolenoidRefNum Registry Set.vi"("refnum name"="Right shift", "SolenoidDevRef"=w80) -> ()  [unwired: 8 in, 2 out]
  n112 = call <vilib>:"WPI_DigitalInputRefNum Registry Set.vi"("error in (no error)"=w36, "refnum name"="Bridge Actuator Down", "DigitalInputDevRef"=w38) -> ()  [unwired: 7 in, 2 out]
  n113 = call <vilib>:"WPI_RelayRefNum Registry Set.vi"("refnum name"="Compressor", "RelayDevRef"=w51) -> ()  [unwired: 8 in, 2 out]
  n114 = call <vilib>:"WPI_ServoOpen.vi"("PWM Channel"=FPGA_DIOPWMChannel."PWM 10", "Digital Module (Module 1)"=FPGA_TypedefDigitalModule."Digital Module 1" ("DIO Module (Slot 4)")) -> ("error out"=w33:errorcluster, "ServoDeviceRef"=w32:T44)  [unwired: 2 in, 6 out]
  n115 = call-poly <vilib>:"WPI_MotorControlOpen.vi"("PWM Channel"=FPGA_DIOPWMChannel."PWM 3", "Digital Module (Module 1)"=FPGA_TypedefDigitalModule."Digital Module 1") -> ("MotorControlDeviceRef"=w143:T26)  [unwired: 8 in, 1 out]
  n116 = disable-structure shown="Disabled" {
    frame Disabled {
      n117 = call <vilib>:"WPI_DigitalInputOpen.vi"("DIO Channel"=FPGA_DIOChannel."DIO 2", "Digital Module (Module 1)"=FPGA_TypedefDigitalModule."Digital Module 1") -> ("DigitalInputDevRef"=w299:T24)  [unwired: 8 in, 1 out]
      n118 = call <vilib>:"WPI_DigitalInputOpen.vi"("DIO Channel"=FPGA_DIOChannel."DIO 3", "Digital Module (Module 1)"=FPGA_TypedefDigitalModule."Digital Module 1") -> ("DigitalInputDevRef"=w295:T24)  [unwired: 8 in, 1 out]
      n119 = call <vilib>:"WPI_DigitalInputRefNum Registry Set.vi"("refnum name"="ball speed front", "DigitalInputDevRef"=w299) -> ()  [unwired: 8 in, 2 out]
      n120 = call <vilib>:"WPI_DigitalInputRefNum Registry Set.vi"("refnum name"="ball speed back", "DigitalInputDevRef"=w295) -> ()  [unwired: 8 in, 2 out]
    }
    frame Enabled {
    }
  }
  n121 = call-poly <vilib>:"WPI_MotorControlOpen.vi"("PWM Channel"=FPGA_DIOPWMChannel."PWM 4", "Digital Module (Module 1)"=FPGA_TypedefDigitalModule."Digital Module 1") -> ("MotorControlDeviceRef"=w138:T26)  [unwired: 8 in, 1 out]
  n122 = call <vilib>:"WPI_DigitalInputOpen.vi"("DIO Channel"=FPGA_DIOChannel."DIO 14", "Digital Module (Module 1)"=FPGA_TypedefDigitalModule."Digital Module 1") -> ("DigitalInputDevRef"=w77:T24)  [unwired: 8 in, 1 out]
  n123 = call <vilib>:"WPI_ServoRefNum Registry Set.vi"("error in (no error)"=w33, "refnum name"="Bridge Lock Servo", "ServoDeviceRef"=w32) -> ()  [unwired: 9 out]
  n124 = call <vilib>:"WPI_MotorControlRefNum Registry Set.vi"("refnum name"="Shooter", "MotorControlDevRef"=w143) -> ()  [unwired: 8 in, 2 out]
  n125 = call <vilib>:"WPI_DigitalInputRefNum Registry Set.vi"("refnum name"="Prime Break Beam", "DigitalInputDevRef"=w77) -> ()  [unwired: 8 in, 2 out]
  n126 = call <vilib>:"WPI_MotorControlRefNum Registry Set.vi"("refnum name"="Turret", "MotorControlDevRef"=w138) -> ()  [unwired: 8 in, 2 out]
  n127 = call <vilib>:"WPI_GyroOpen.vi"("Analog Channel"=FPGA_AIGyroChannel."AI 2", "Analog Module (Module 1)"=FPGA_TypedefAnalogModuleForGyro."Analog Module 1") -> ("error out"=w8:errorcluster, "GyroDevRef"=w4:T37)  [unwired: 7 in, 1 out]
  n128 = call <vilib>:"WPI_RelayOpen.vi"("Relay Direction"=WPI_RelayDirection."Both directions", "Relay Channel"=FPGA_DIORelayChannel."Relay 8", "Digital Module (Module 1)"=FPGA_TypedefDigitalModule."Digital Module 1" ("Relay Digital Module (Module 1)")) -> ("RelayDevRef"=w9:T21)  [unwired: 7 in, 1 out]
  n129 = call-poly <vilib>:"WPI_MotorControlOpen.vi"("PWM Channel"=FPGA_DIOPWMChannel."PWM 5", "Digital Module (Module 1)"=FPGA_TypedefDigitalModule."Digital Module 1") -> ("MotorControlDeviceRef"=w124:T26)  [unwired: 8 in, 1 out]
  n130 = call-poly <vilib>:"WPI_MotorControlOpen.vi"("Invert"=TRUE, "PWM Channel"=FPGA_DIOPWMChannel."PWM 6", "Digital Module (Module 1)"=FPGA_TypedefDigitalModule."Digital Module 1") -> ("MotorControlDeviceRef"=w127:T26)  [unwired: 7 in, 1 out]
  n131 = call-poly <vilib>:"WPI_MotorControlOpen.vi"("Invert"=TRUE, "PWM Channel"=FPGA_DIOPWMChannel."PWM 7", "Digital Module (Module 1)"=FPGA_TypedefDigitalModule."Digital Module 1") -> ("MotorControlDeviceRef"=w60:T26)  [unwired: 7 in, 1 out]
  n132 = call <vilib>:"WPI_GyroSetGain.vi"("error in (no error)"=w8, "Gain (VoltsPerDegree/Second)"=0.00608, "GyroDevRef"=w4) -> ("error out"=w7:errorcluster, "GyroDevRef"=w5:T37)  [unwired: 7 in]
  n133 = call <vilib>:"WPI_RelaySet.vi"("RelayValue"=WPI_RelayValue."Off", "RelayDevRef"=w9) -> ("RelayDevRef"=w10:T21)  [unwired: 8 in, 1 out]
  n134 = call <vilib>:"WPI_MotorControlRefNum Registry Set.vi"("refnum name"="Intake", "MotorControlDevRef"=w124) -> ()  [unwired: 8 in, 2 out]
  n135 = call <vilib>:"WPI_MotorControlRefNum Registry Set.vi"("refnum name"="Fire Conveyor", "MotorControlDevRef"=w127) -> ()  [unwired: 8 in, 2 out]
  n136 = call <vilib>:"WPI_MotorControlRefNum Registry Set.vi"("refnum name"="Middle Conveyor", "MotorControlDevRef"=w60) -> ()  [unwired: 8 in, 2 out]
  n137 = call <vilib>:"WPI_RelayRefNum Registry Set.vi"("refnum name"="Sonar Kick", "RelayDevRef"=w10) -> ()  [unwired: 8 in, 2 out]
  n138 = call <vilib>:"WPI_GyroRefNum Registry Set.vi"("error in (no error)"=w7, "refnum name"="Pitch Gyro", "GyroDevRef"=w5) -> ()  [unwired: 7 in, 2 out]
  n139 = call-poly <vilib>:"WPI_MotorControlOpen.vi"("Invert"=TRUE, "PWM Channel"=FPGA_DIOPWMChannel."PWM 8", "Digital Module (Module 1)"=FPGA_TypedefDigitalModule."Digital Module 1") -> ("MotorControlDeviceRef"=w55:T26)  [unwired: 7 in, 1 out]
  n140 = call <vilib>:"WPI_MotorControlRefNum Registry Set.vi"("refnum name"="Lower Conveyor", "MotorControlDevRef"=w55) -> ()  [unwired: 8 in, 2 out]
